vi "temperature.vi"() -> ()   [LabVIEW 2015]
uses:
  Enum_pomiar_temp.ctl
  <vilib>/DAQmx/read.llb/DAQmx Read (Analog DBL 1Chan 1Samp).vi
  <vilib>/DAQmx/create/channels.llb/DAQmx Create Channel (AI-Voltage-Basic).vi
  <vilib>/DAQmx/configure/timing.llb/DAQmx Timing (Sample Clock).vi
  <vilib>/DAQmx/miscellaneous.llb/DAQmx Fill In Error Info.vi
panel:
  out "Thermometer":dbl(slide) scale=0.0..100.0
  out "Numeric":dbl
  in  "DAQmx Physical Channel":tag
  in  "stop":bool
  in  "Boolean":bool
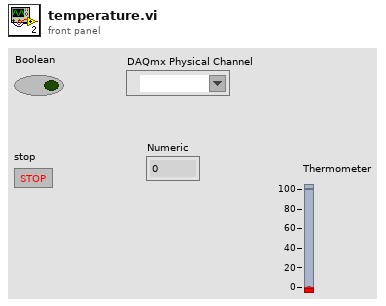
[diagram p1: front panel]
types:
  T1 = typedef "Enum_pomiar_temp.ctl" = enum16{"Init", "Pomiar", "STOP", "Wait for events", "Zapis"}
  T2 = enum16{"open", "replace", "create", "open or create", "replace or create", "replace or create with confirmation"}
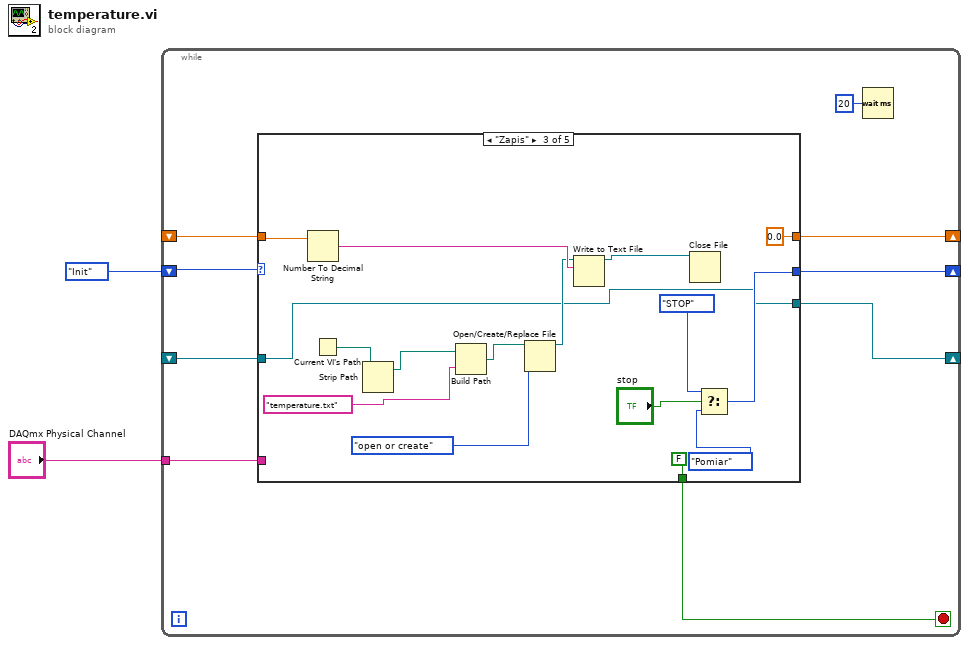
[diagram p0: block diagram]
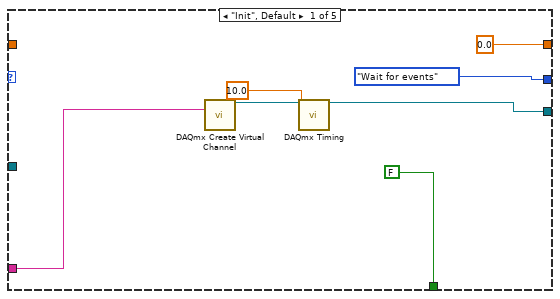
[diagram p2: hidden frame]
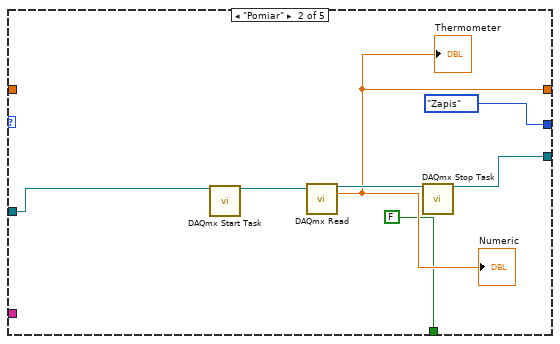
[diagram p3: hidden frame]
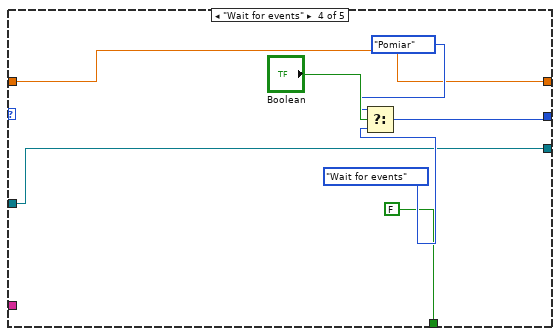
[diagram p4: hidden frame]
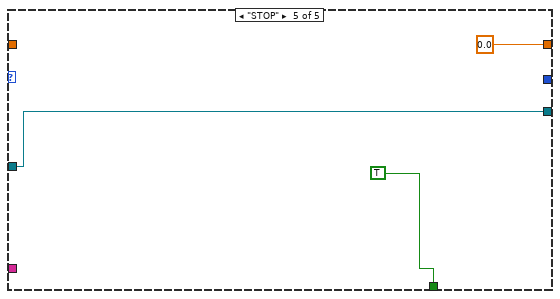
[diagram p5: hidden frame]
diagram:
  n1 = while {
    shift-right: [w6] -> _
    shift-left: Enum_pomiar_temp."Init" -> [w11]
    shift-right: [w8] -> _
    shift-left: _ -> [w7]
    tunnel: "DAQmx Physical Channel" -> [w9]
    shift-right: [w5] -> _
    shift-left: _ -> [w4]
    stop <- w3 stop-if-true
    n2 = case shown="\"Zapis\"" w11 {
      tunnel: w9 -> [w17 _ _ _ _]
      tunnel: [w15 w22 w30 w45 w49] -> w8
      tunnel: w7 -> [_ w25 w30 w45 w49]
      tunnel: [Enum_pomiar_temp."Wait for events" Enum_pomiar_temp."Zapis" w32 w42 _] -> w6
      tunnel: [0.0 ("data") w20 0.0 ("data") w44 0.0 ("data")] -> w5
      tunnel: w4 -> [_ _ w41 w44 _]
      tunnel: [FALSE FALSE FALSE FALSE TRUE] -> w3
      frame "Init", Default {
        n3 = call-poly <vilib>:"DAQmx Create Virtual Channel.vi"("physical channels"=w17) -> ("task out"=w18:refnum<k21>)  [unwired: 13 in, 1 out]
        n4 = call-poly <vilib>:"DAQmx Timing.vi"("task/channels in"=w18, "rate"=10.0) -> ("task out"=w15:refnum<k21>)  [unwired: 12 in, 1 out]
      }
      frame "Pomiar" {
        n5 = call <vilib>:"DAQmx Start Task.vi"("task/channels in"=w25) -> ("task out"=w24:refnum<k21>)  [unwired: 13 in, 1 out]
        n6 = call-poly <vilib>:"DAQmx Read.vi"("task/channels in"=w24) -> ("task out"=w23:refnum<k21>, "data"=w20:dbl)  [unwired: 12 in, 1 out]
        "Numeric" <- w20
        "Thermometer" <- w20
        n7 = call <vilib>:"DAQmx Stop Task.vi"("task/channels in"=w23) -> ("task out"=w22:refnum<k21>)  [unwired: 13 in, 1 out]
      }
      frame "Zapis" {
        n8 = Number To Decimal String(number=w41) -> (decimal integer string=w40:string)  [unwired: 1 in]
        n9 = Current VI's Path() -> (path=w28:path)
        n10 = Strip Path(path=w28) -> (stripped path=w27:path)  [unwired: 1 out]
        n11 = Build Path(base path=w27, name or relative path="temperature.txt") -> (appended path=w39:path)
        n12 = Open/Create/Replace File(file path (use dialog)=w39, operation (0:open)=T2."open or create") -> (refnum out=w38:refnum<file>)  [unwired: 4 in, 2 out]
        n13 = Write to Text File(file (use dialog)=w38, text=w40) -> (refnum out=w37:refnum<file>)  [unwired: 2 in, 2 out]
        n14 = Close File(refnum=w37) -> ()  [unwired: 1 in, 2 out]
        n15 = Select(t=Enum_pomiar_temp."STOP", s="stop", f=Enum_pomiar_temp."Pomiar") -> (s? t:f=w32:T1)
      }
      frame "Wait for events" {
        n16 = Select(t=Enum_pomiar_temp."Pomiar", s="Boolean", f=Enum_pomiar_temp."Wait for events") -> (s? t:f=w42:T1)
      }
      frame "STOP" {
      }
    }
    n17 = Wait (ms)(milliseconds to wait=u32 20) -> ()  [unwired: 1 out]
  }
